vi "Teleop.vi"(10 "Match Info":T1={"Autonomous Elapsed Seconds"=0.0, "TeleOp Elapsed Seconds"=0.0, "Disabled Elapsed Seconds"=0.0, "Visited Autonomous"=FALSE, "Visited TeleOp"=FALSE, "Visited Disabled"=FALSE, "Autonomous Settings"={"Autonomous Style"=enum."Independent", "VI Refnum"=refnum}}, 11 "Call Context":T2) -> ()   [LabVIEW 2016]
doc: "This VI is called for each TeleOp packet received from the DS where the robot is not disabled. It is often used to read from the joysticks and update I/O or to update setpoints for timed control loops. It should complete and return within 20 milliseconds or it may miss DS packets."
uses:
  <vilib>/Rock Robotics/WPI/DriverStation/WPI_DriverStationDerivedRobotMode.ctl
  <vilib>/Rock Robotics/WPI/DriverStation/WPI_DriverStationMatch Info.ctl
  <vilib>/Rock Robotics/Network Tables/NT Read Boolean.vi
  <vilib>/Rock Robotics/Network Tables/NT Read Number.vi
  <vilib>/Rock Robotics/WPI/Utilities/WPI_GetSetVariantRefNum.vi
  <vilib>/Rock Robotics/Network Tables/NT Write Numeric Array.vi
  <vilib>/Rock Robotics/Network Tables/NT Write Boolean Array.vi
panel:
  out "Test Button 2":dbl
  out "Test Button 1":dbl
  out "Test2":dbl
  out "Test1":dbl
  out "Lift Bottom":dbl
  out "Lift Top":dbl
  out "Sample Slider 0":dbl(slide) scale=0.0..5.0
  out "Sample Boolean 1":bool
  out "Sample Boolean 0":bool
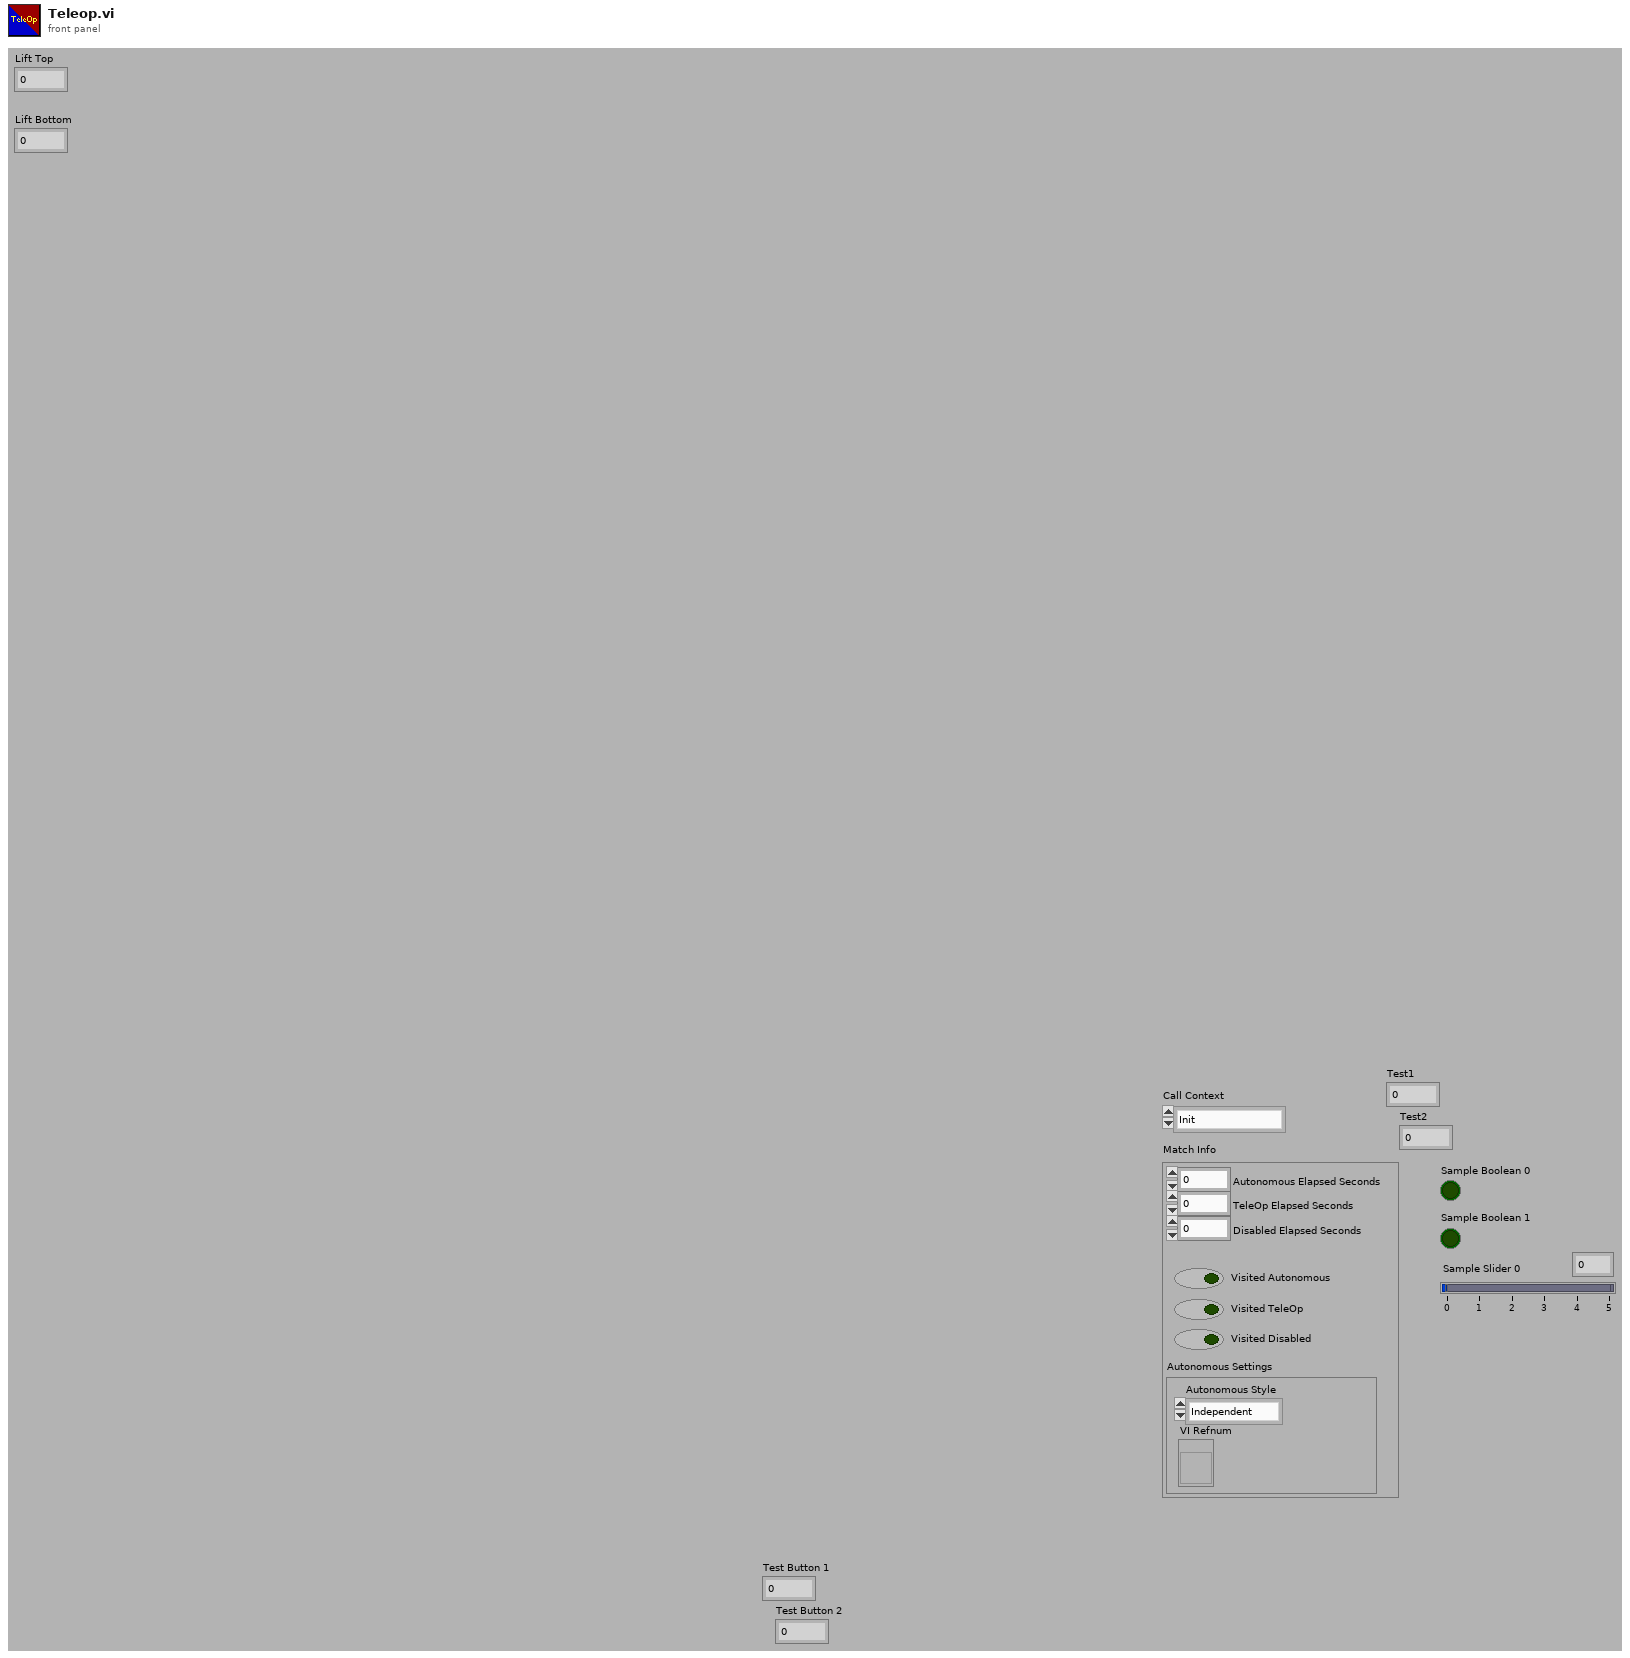
[diagram p1: front panel]
types:
  T1 = typedef "WPI_DriverStationMatch Info.ctl" = cluster{"Autonomous Elapsed Seconds":dbl, "TeleOp Elapsed Seconds":dbl, "Disabled Elapsed Seconds":dbl, "Visited Autonomous":bool, "Visited TeleOp":bool, "Visited Disabled":bool, "Autonomous Settings":cluster{"Autonomous Style":enum16{"Iterative", "Independent"}, "VI Refnum":refnum<vi>}}
  T2 = typedef "WPI_DriverStationDerivedRobotMode.ctl" = enum16{"Init", "Execute", "Stop"}
  T3 = typedef "WPI_MotorControlDeviceRef.ctl" = cluster{"DeviceStatus":errorcluster, "Type":T4, "PWM":cluster{"PWM Channel":T5, "DeadBand":T6}, "CAN":cluster{"Device Number":u8, "SetOutput VI Ref":variant, "GetOutput VI Ref":variant, "Enable VI Ref":variant, "Disable VI Ref":variant, "Data":variant}, "Invert":bool}
  T4 = typedef "WPI_MotorControlType.ctl" = enum16{"PWM", "CAN"}
  T5 = typedef "FPGA_DIOPWMChannel.ctl" = enum8{"PWM 0", "PWM 1", "PWM 2", "PWM 3", "PWM 4", "PWM 5", "PWM 6", "PWM 7", "PWM 8", "PWM 9", "PWM MXP 0", "PWM MXP 1", "PWM MXP 2", "PWM MXP 3", "PWM MXP 4", "PWM MXP 5", "PWM MXP 6", "PWM MXP 7", "PWM MXP 8", "PWM MXP 9", "Invalid"}
  T6 = typedef "WPI_PWMDeadband.ctl" = cluster{"Name":string, "maxPositivePwm":i32, "minPositivePwm":i32, "centerPwm":i32, "maxNegativePwm":i32, "minNegativePwm":i32, "angularRange":u16}
  T7 = typedef "WPI_JoystickDevRef.ctl" = cluster{"Device":T8}
  T8 = typedef "WPI_JoystickDeviceEnum.ctl" = enum16{"USB 0", "USB 1", "USB 2", "USB 3", "USB 4", "USB 5"}
  T9 = cluster{"Buttons[0]":bool, "Buttons[1]":bool, "Buttons[2]":bool, "Buttons[3]":bool, "Buttons[4]":bool, "Buttons[5]":bool, "Buttons[6]":bool, "Buttons[7]":bool, "Buttons[8]":bool}
  T10 = typedef "WPI_DigitalInputDevRef.ctl" = cluster{"DevStatus":errorcluster, "DIO Channel":T11}
  T11 = typedef "FPGA_DIOChannel.ctl" = enum8{"DIO 0", "DIO 1", "DIO 2", "DIO 3", "DIO 4", "DIO 5", "DIO 6", "DIO 7", "DIO 8", "DIO 9", "DIO MXP 0", "DIO MXP 1", "DIO MXP 2", "DIO MXP 3", "DIO MXP 4", "DIO MXP 5", "DIO MXP 6", "DIO MXP 7", "DIO MXP 8", "DIO MXP 9", "DIO MXP 10", "DIO MXP 11", "DIO MXP 12", "DIO MXP 13", "DIO MXP 14", "DIO MXP 15", "SPI Port CS1", "SPI Port CS2", "SPI Port CS3", "SPI Port MISO", "SPI Port MOSI", "Invalid"}
  T12 = typedef "WPI_RobotDriveDevRef.ctl" = cluster{"DevStatus":errorcluster, "Motors[]":T3[], "Square Inputs":bool, "Max Output":dbl}
  T13 = cluster{"Axes[0]":dbl, "Axes[1]":dbl, "Axes[2]":dbl, "Axes[3]":dbl, "Axes[4]":dbl, "Axes[5]":dbl, "Axes[6]":dbl, "Axes[7]":dbl, "Axes[8]":dbl}
  T14 = typedef "WPI_ServoDeviceRef.ctl" = cluster{"DeviceStatus":errorcluster, "PWM Channel":T5, "DeadBand":T6}
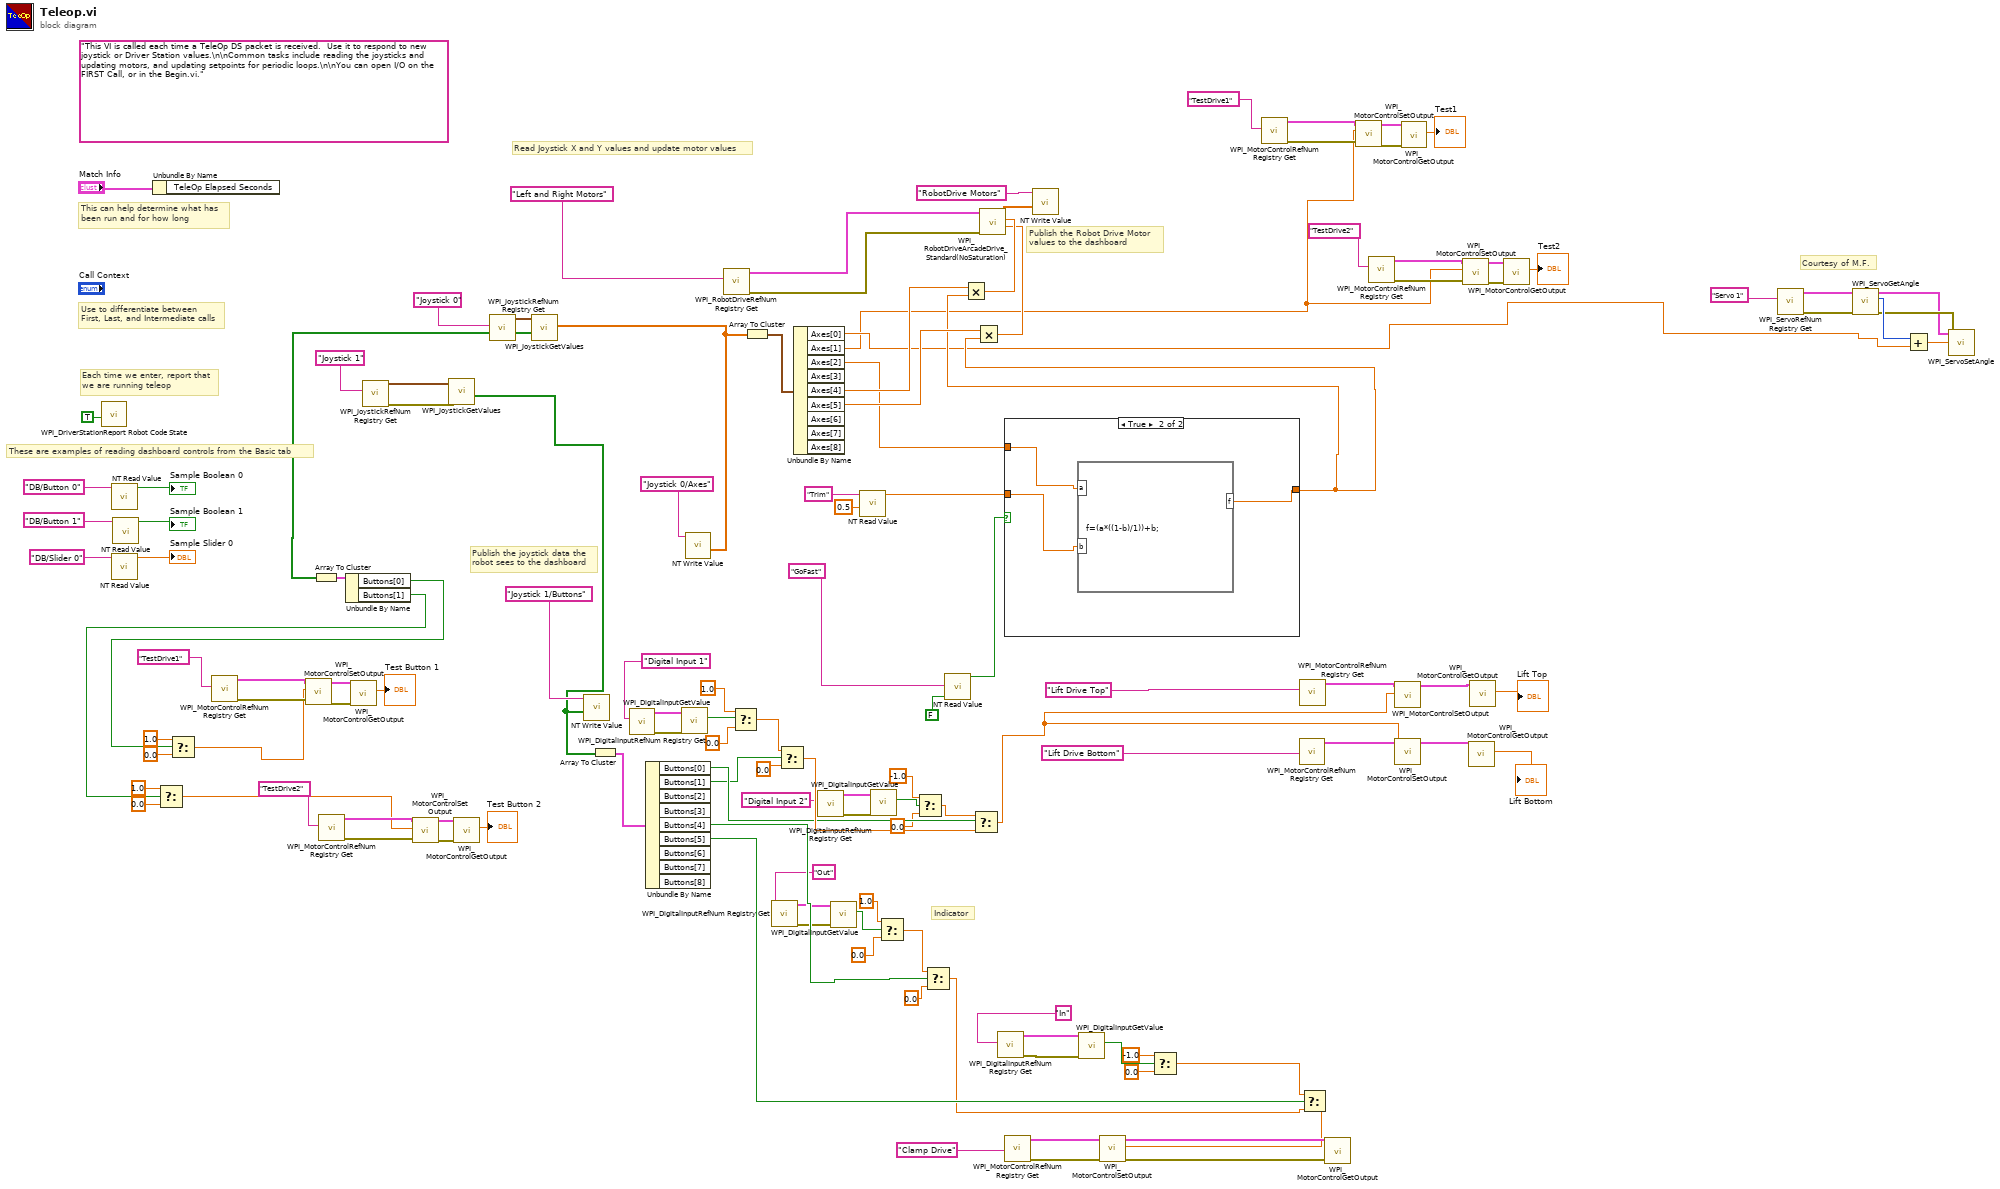
[diagram p0: block diagram]
diagram:
  (unwired) "This VI is called each time a TeleOp DS packet is received.  Use it to respond to new joystick or Driver Station values.\n\nCommon tasks include reading the joysticks and updating motors, and updating setpoints for periodic loops.\n\nYou can open I/O on the FIRST Call, or in the Begin.vi."
  # "Courtesy of M.F."
  # "Indicator"
  # "Publish the Robot Drive Motor\nvalues to the dashboard"
  # "Publish the joystick data the\nrobot sees to the dashboard"
  # "Read Joystick X and Y values and update motor values"
  # "These are examples of reading dashboard controls from the Basic tab"
  # "Each time we enter, report that\nwe are running teleop"
  # "Use to differentiate between\nFirst, Last, and Intermediate calls"
  # "This can help determine what has\nbeen run and for how long"
  n1 = call <vilib>:"WPI_DriverStationReport Robot Code State.vi"("TeleOp"=TRUE ("Autonomous")) -> ()  [unwired: 10 in, 1 out]
  n2 = call-poly <vilib>:"NT Read Value.vi"("Name"="DB/Button 0" ("refnum name")) -> ("Boolean"=→"Sample Boolean 0":bool)  [unwired: 9 in, 1 out]
  n3 = call-poly <vilib>:"NT Read Value.vi"("Name"="DB/Slider 0" ("refnum name")) -> ("Numeric"=→"Sample Slider 0":dbl)  [unwired: 9 in, 1 out]
  n4 = call-poly <vilib>:"NT Read Value.vi"("Name"="DB/Button 1" ("refnum name")) -> ("Boolean"=→"Sample Boolean 1":bool)  [unwired: 9 in, 1 out]
  n5 = Unbundle By Name("Match Info") -> ()  [unwired: 1 out]
  n6 = call <vilib>:"WPI_MotorControlRefNum Registry Get.vi"("refnum name"="TestDrive1") -> ("error out"=w15:errorcluster, "MotorControlDevRef"=w22:T3)  [unwired: 9 in]
  n7 = call <vilib>:"WPI_MotorControlRefNum Registry Get.vi"("refnum name"="TestDrive2") -> ("error out"=w14:errorcluster, "MotorControlDevRef"=w19:T3)  [unwired: 9 in]
  n8 = call <vilib>:"WPI_JoystickRefNum Registry Get.vi"("refnum name"="Joystick 1") -> ("error out"=w37:errorcluster, "JoystickDevRef"=w81:T7)  [unwired: 9 in]
  n9 = call <vilib>:"WPI_JoystickGetValues.vi"("error in (no error)"=w37, "JoystickDevRef"=w81) -> ("Buttons"=w80:bool[])  [unwired: 5 in, 4 out]
  n10 = call <vilib>:"WPI_JoystickRefNum Registry Get.vi"("refnum name"="Joystick 0") -> ("JoystickDevRef"=w120:T7)  [unwired: 1 in, 9 out]
  n11 = call <vilib>:"WPI_JoystickGetValues.vi"("JoystickDevRef"=w120) -> ("Buttons"=w10:bool[], "Axes"=w95:dbl[])  [unwired: 6 in, 3 out]
  n12 = Array To Cluster(array=w10) -> (cluster=w9:T9)
  n13 = Unbundle By Name(w9) -> ("Buttons[0]"=w8:bool, "Buttons[1]"=w7:bool)
  n14 = Select(t=1.0, s=w7, f=0.0) -> (s? t:f=w4:dbl)
  n15 = Select(t=1.0, s=w8, f=0.0) -> (s? t:f=w3:dbl)
  n16 = call <vilib>:"WPI_MotorControlSetOutput.vi"("error in (no error)"=w15, "Output"=w3, "MotorControlDevRef"=w22) -> ("error out"=w13:errorcluster, "MotorControlDevRef"=w18:T3)  [unwired: 6 in, 1 out]
  n17 = call <vilib>:"WPI_MotorControlGetOutput.vi"("error in"=w13, "MotorControlDevRef"=w18) -> ("Output"=→"Test Button 1":dbl)  [unwired: 7 in, 2 out]
  n18 = call <vilib>:"WPI_MotorControlSetOutput.vi"("error in (no error)"=w14, "Output"=w4, "MotorControlDevRef"=w19) -> ("error out"=w11:errorcluster, "MotorControlDevRef"=w16:T3)  [unwired: 6 in, 1 out]
  n19 = call <vilib>:"WPI_MotorControlGetOutput.vi"("error in"=w11, "MotorControlDevRef"=w16) -> ("Output"=→"Test Button 2":dbl)  [unwired: 7 in, 2 out]
  n20 = call-poly <vilib>:"NT Write Value.vi"("Boolean Array"=w80, "Name"="Joystick 1/Buttons") -> ()  [unwired: 9 in, 1 out]
  n21 = Array To Cluster(array=w80) -> (cluster=w96:T9)
  n22 = call <vilib>:"WPI_DigitalInputRefNum Registry Get.vi"("refnum name"="Digital Input 1") -> ("error out"=w62:errorcluster, "DigitalInputDevRef"=w63:T10)  [unwired: 9 in]
  n23 = Unbundle By Name(w96) -> ("Buttons[0]"=w82:bool, "Buttons[1]"=w59:bool, "Buttons[4]"=w56:bool, "Buttons[5]"=w58:bool)  [unwired: 5 out]
  n24 = call <vilib>:"WPI_DigitalInputGetValue.vi"("error in (no error)"=w62, "DigitalInputDevRef"=w63) -> ("Value"=w61:bool)  [unwired: 7 in, 2 out]
  n25 = call-poly <vilib>:"NT Write Value.vi"("Numeric Array"=w95, "Name"="Joystick 0/Axes") -> ()  [unwired: 9 in, 1 out]
  n26 = call <vilib>:"WPI_RobotDriveRefNum Registry Get.vi"("refnum name"="Left and Right Motors") -> ("error out"=w91:errorcluster, "RobotDriveDevRef"=w121:T12)  [unwired: 1 in, 8 out]
  n27 = Select(t=1.0, s=w61, f=0.0) -> (s? t:f=w72:dbl)
  n28 = Array To Cluster(array=w95) -> (cluster=w94:T13)
  n29 = call <vilib>:"WPI_DigitalInputRefNum Registry Get.vi"("refnum name"="Out") -> ("error out"=w46:errorcluster, "DigitalInputDevRef"=w55:T10)  [unwired: 9 in]
  n30 = Select(t=w72, s=w59, f=0.0) -> (s? t:f=w102:dbl)
  n31 = Unbundle By Name(w94) -> ("Axes[0]"=w36:dbl, "Axes[1]"=w23:dbl, "Axes[2]"=w83:dbl, "Axes[4]"=w93:dbl, "Axes[5]"=w92:dbl)  [unwired: 4 out]
  n32 = call <vilib>:"WPI_DigitalInputRefNum Registry Get.vi"("refnum name"="Digital Input 2") -> ("error out"=w66:errorcluster, "DigitalInputDevRef"=w67:T10)  [unwired: 9 in]
  n33 = call <vilib>:"WPI_DigitalInputGetValue.vi"("error in (no error)"=w46, "DigitalInputDevRef"=w55) -> ("Value"=w53:bool)  [unwired: 7 in, 2 out]
  n34 = call-poly <vilib>:"NT Read Value.vi"("Default Value"=0.5, "Name"="Trim" ("refnum name")) -> ("Numeric"=w87:dbl)  [unwired: 8 in, 1 out]
  n35 = call <vilib>:"WPI_DigitalInputGetValue.vi"("error in (no error)"=w66, "DigitalInputDevRef"=w67) -> ("Value"=w65:bool)  [unwired: 7 in, 2 out]
  n36 = Select(t=1.0, s=w53, f=0.0) -> (s? t:f=w50:dbl)
  n37 = Select(t=-1.0, s=w65, f=0.0) -> (s? t:f=w73:dbl)
  n38 = Select(t=w50, s=w56, f=0.0) -> (s? t:f=w47:dbl)
  n39 = call-poly <vilib>:"NT Read Value.vi"("Default Value"=FALSE, "Name"="GoFast" ("refnum name")) -> ("Boolean"=w89:bool)  [unwired: 8 in, 1 out]
  n40 = Select(t=w73, s=w82, f=w102) -> (s? t:f=w103:dbl)
  n41 = call <vilib>:"WPI_DigitalInputRefNum Registry Get.vi"("refnum name"="In") -> ("error out"=w77:errorcluster, "DigitalInputDevRef"=w79:T10)  [unwired: 9 in]
  n42 = case shown="True" w89 {
    tunnel: [w131 w132] -> w85
    tunnel: w87 -> [w131 w133]
    tunnel: w83 -> [_ w134]
    frame False {
    }
    frame True {
      n43 = formula code="f=(a*((1-b)/1))+b;"("a"=w134, "b"=w133) -> ("f"=w132:dbl)
    }
  }
  n44 = Multiply(x=w93, y=w85) -> (x*y=w113:dbl)
  n45 = Multiply(x=w92, y=w85) -> (x*y=w112:dbl)
  n46 = call <vilib>:"WPI_RobotDriveArcadeDrive_Standard(NoSaturation).vi"("error in (no error)"=w91, "Y axis value"=w112, "X axis value"=w113, "RobotDriveDevRef"=w121) -> ("Motor Values"=w116:dbl[])  [unwired: 7 out]
  n47 = call <vilib>:"WPI_MotorControlRefNum Registry Get.vi"("refnum name"="Clamp Drive") -> ("error out"=w101:errorcluster, "MotorControlDevRef"=w99:T3)  [unwired: 9 in]
  n48 = call-poly <vilib>:"NT Write Value.vi"("Numeric Array"=w116, "Name"="RobotDrive Motors") -> ()  [unwired: 9 in, 1 out]
  n49 = call <vilib>:"WPI_DigitalInputGetValue.vi"("error in (no error)"=w77, "DigitalInputDevRef"=w79) -> ("Value"=w75:bool)  [unwired: 7 in, 2 out]
  n50 = Select(t=-1.0, s=w75, f=0.0) -> (s? t:f=w48:dbl)
  n51 = call <vilib>:"WPI_MotorControlRefNum Registry Get.vi"("refnum name"="TestDrive1") -> ("error out"=w28:errorcluster, "MotorControlDevRef"=w35:T3)  [unwired: 9 in]
  n52 = call <vilib>:"WPI_MotorControlRefNum Registry Get.vi"("refnum name"="Lift Drive Bottom") -> ("MotorControlDevRef"=w108:T3)  [unwired: 9 in, 1 out]
  n53 = call <vilib>:"WPI_MotorControlRefNum Registry Get.vi"("refnum name"="Lift Drive Top") -> ("MotorControlDevRef"=w109:T3)  [unwired: 9 in, 1 out]
  n54 = Select(t=w48, s=w58, f=w47) -> (s? t:f=w74:dbl)
  n55 = call <vilib>:"WPI_MotorControlSetOutput.vi"("error in (no error)"=w101, "Output"=w74, "MotorControlDevRef"=w99) -> ("error out"=w98:errorcluster, "MotorControlDevRef"=w100:T3)  [unwired: 6 in, 1 out]
  n56 = call <vilib>:"WPI_MotorControlGetOutput.vi"("error in"=w98, "MotorControlDevRef"=w100) -> ()  [unwired: 7 in, 3 out]
  n57 = call <vilib>:"WPI_MotorControlSetOutput.vi"("error in (no error)"=w28, "Output"=w23, "MotorControlDevRef"=w35) -> ("error out"=w26:errorcluster, "MotorControlDevRef"=w31:T3)  [unwired: 6 in, 1 out]
  n58 = call <vilib>:"WPI_MotorControlRefNum Registry Get.vi"("refnum name"="TestDrive2") -> ("error out"=w27:errorcluster, "MotorControlDevRef"=w32:T3)  [unwired: 9 in]
  n59 = call <vilib>:"WPI_MotorControlSetOutput.vi"("Output"=w103, "MotorControlDevRef"=w109) -> ("MotorControlDevRef"=w110:T3)  [unwired: 7 in, 2 out]
  n60 = call <vilib>:"WPI_MotorControlSetOutput.vi"("Output"=w103, "MotorControlDevRef"=w108) -> ("MotorControlDevRef"=w111:T3)  [unwired: 7 in, 2 out]
  n61 = call <vilib>:"WPI_MotorControlGetOutput.vi"("error in"=w26, "MotorControlDevRef"=w31) -> ("Output"=→"Test1":dbl)  [unwired: 7 in, 2 out]
  n62 = call <vilib>:"WPI_MotorControlSetOutput.vi"("error in (no error)"=w27, "Output"=w23, "MotorControlDevRef"=w32) -> ("error out"=w24:errorcluster, "MotorControlDevRef"=w29:T3)  [unwired: 6 in, 1 out]
  n63 = call <vilib>:"WPI_MotorControlGetOutput.vi"("MotorControlDevRef"=w111) -> ("Output"=→"Lift Bottom":dbl)  [unwired: 8 in, 2 out]
  n64 = call <vilib>:"WPI_MotorControlGetOutput.vi"("MotorControlDevRef"=w110) -> ("Output"=→"Lift Top":dbl)  [unwired: 8 in, 2 out]
  n65 = call <vilib>:"WPI_MotorControlGetOutput.vi"("error in"=w24, "MotorControlDevRef"=w29) -> ("Output"=→"Test2":dbl)  [unwired: 7 in, 2 out]
  n66 = call <vilib>:"WPI_ServoRefNum Registry Get.vi"("refnum name"="Servo 1") -> ("error out"=w41:errorcluster, "ServoDeviceRef"=w42:T14)  [unwired: 9 in]
  n67 = call <vilib>:"WPI_ServoGetAngle.vi"("ServoDeviceRef"=w42, "error in (no error)"=w41) -> ("ServoDeviceRef"=w39:T14, "Angle"=w44:u16, "error out"=w40:errorcluster)  [unwired: 6 in]
  n68 = Add(x=w44, y=w36) -> (x+y=w45:dbl)
  n69 = call <vilib>:"WPI_ServoSetAngle.vi"("error in (no error)"=w40, "Angle"=w45, "ServoDeviceRef"=w39) -> ()  [unwired: 7 in, 2 out]
